vi "panelResize.vi"(4 "error in (no error)":errorcluster, 5 "NewBnds":T1, 7 "control refs":T2) -> (0 "error out":errorcluster)   [LabVIEW 2017]
uses:
  <vilib>/Utility/miscctls.llb/LVRectTypeDef.ctl
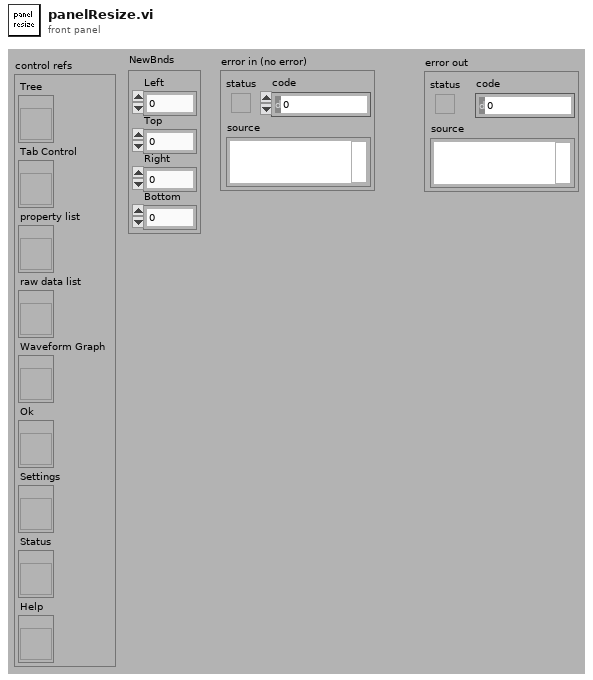
[diagram p1: front panel]
types:
  T1 = typedef "LVRectTypeDef.ctl" = cluster{"Left":i16, "Top":i16, "Right":i16, "Bottom":i16}
  T2 = cluster{"Tree":refnum<vi>, "Tab Control":refnum<vi>, "property list":refnum<vi>, "raw data list":refnum<vi>, "Waveform Graph":refnum<vi>, "Ok":refnum<vi>, "Settings":refnum<vi>, "Status":refnum<vi>, "Help":refnum<vi>}
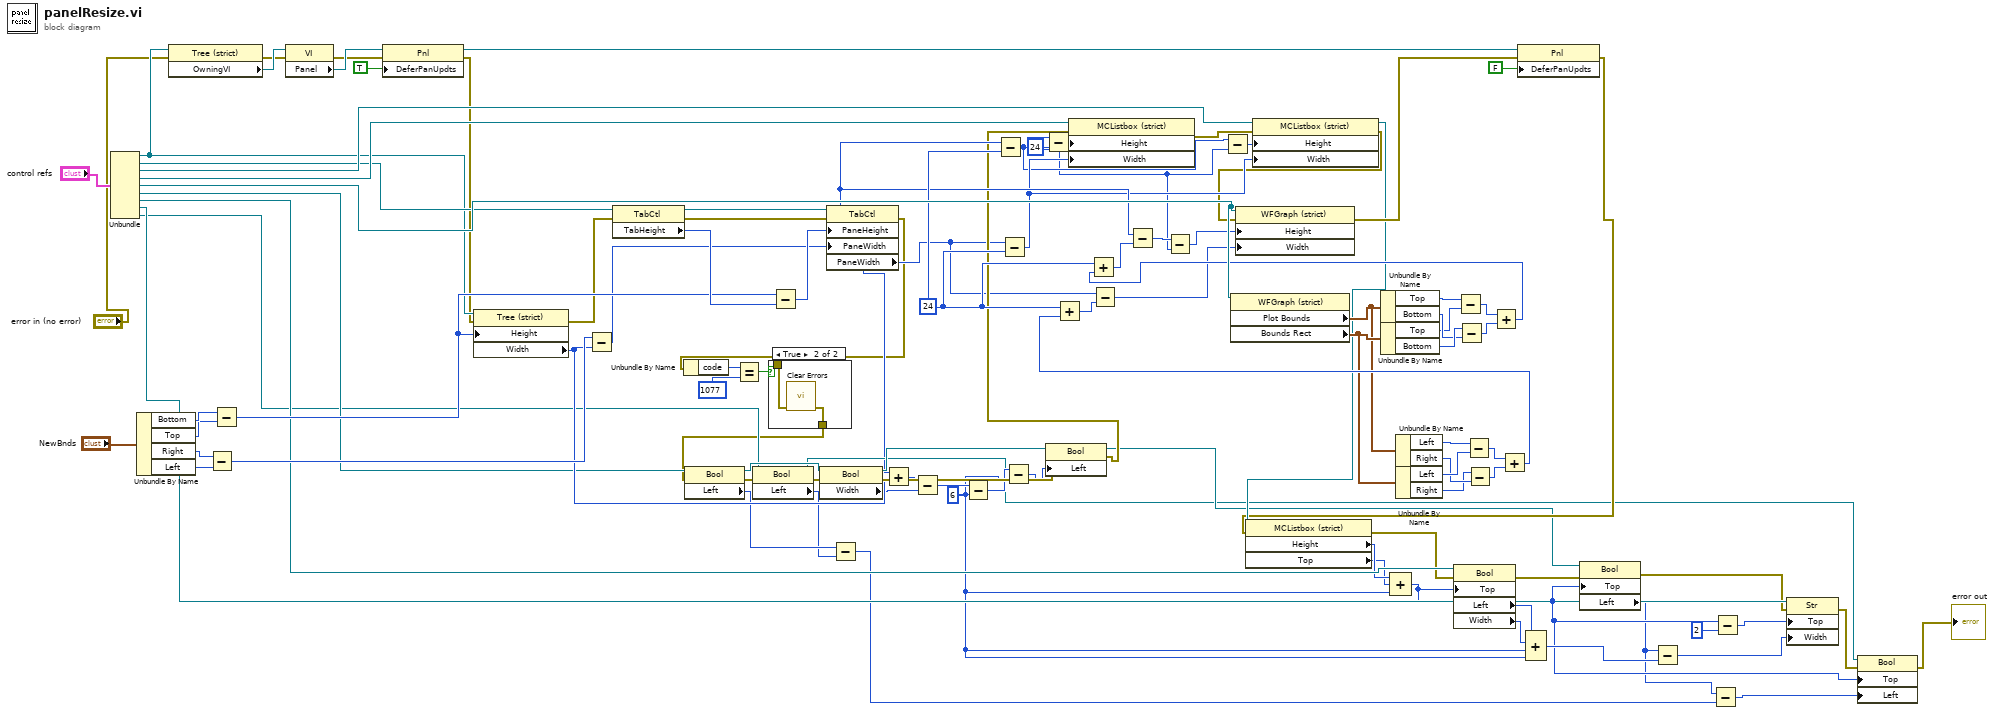
[diagram p0: block diagram]
diagram:
  w42 = u32 24 ("y")
  w23 = u32 6 ("y")
  w92 = u32 24 ("y")
  n1 = Unbundle("control refs") -> ("Tree"=w62:refnum<vi>, "Tab Control"=w101:refnum<vi>, "property list"=w102:refnum<vi>, "raw data list"=w103:refnum<vi>, "Waveform Graph"=w104:refnum<vi>, "Ok"=w22:refnum<vi>, "Settings"=w50:refnum<vi>, "Status"=w33:refnum<vi>, "Help"=w20:refnum<vi>)
  n2 = Unbundle By Name("NewBnds") -> ("Bottom"=w69:i16, "Top"=w68:i16, "Right"=w98:i16, "Left"=w95:i16)
  n3 = property class="Tree (strict)"(reference=w62, error in="error in (no error)") -> (error out=w59:errorcluster, "OwningVI"=w61:refnum<vi>)  [unwired: 1 out]
  n4 = Subtract(x=w98, y=w95) -> (x-y=w96:i16)
  n5 = Subtract(x=w69, y=w68) -> (x-y=w71:i16)
  n6 = property class="VI"(reference=w61, error in=w59) -> (error out=w58:errorcluster, "Panel"=w60:refnum<vi>)  [unwired: 1 out]
  n7 = property class="Pnl"(reference=w60, error in=w58, "DeferPanUpdts"=TRUE ("Defer Panel Updates")) -> (reference out=w54:refnum<vi>, error out=w52:errorcluster)
  n8 = property class="Tree (strict)"(reference=w62, error in=w52, "Height"=w71) -> (error out=w65:errorcluster, "Width"=w51:u32)  [unwired: 1 out]
  n9 = Subtract(x=w96, y=w51) -> (x-y=w7:u32)
  n10 = property class="TabCtl"(reference=w101, error in=w65) -> (reference out=w70:refnum<vi>, error out=w6:errorcluster, "TabHeight"=w72:u32)
  n11 = Subtract(x=w71, y=w72) -> (x-y=w75:u32)
  n12 = property class="TabCtl"(reference=w70, error in=w6, "PaneHeight"=w75, "PaneWidth"=w7) -> (error out=w2:errorcluster, "PaneWidth"=w8:u32)  [unwired: 1 out]
  n13 = Unbundle By Name(w2) -> ("code"=w5:i32)
  n14 = Equal?(x=w5, y=1077) -> (x = y?=w3:bool)
  n15 = case shown="True" w3 {
    tunnel: w2 -> [w105 w107]
    tunnel: [w105 w106] -> w1
    frame False {
    }
    frame True {
      n16 = call <vilib>:"Clear Errors.vi"("error in (no error)"=w107) -> ("error out"=w106:errorcluster)  [unwired: 5 in, 1 out]
    }
  }
  n17 = property class="Bool"(reference=w22, error in=w1) -> (reference out=w21:refnum<vi>, error out=w19:errorcluster, "Left"=w12:i32)
  n18 = property class="Bool"(reference=w20, error in=w19) -> (reference out=w17:refnum<vi>, error out=w18:errorcluster, "Left"=w11:i32)
  n19 = property class="Bool"(reference=w21, error in=w18) -> (reference out=w97:refnum<vi>, error out=w66:errorcluster, "Width"=w48:u32)
  n20 = Subtract(x=w12, y=w11) -> (x-y=w10:i32)
  n21 = Add(x=w8, y=w51) -> (x+y=w49:u32)
  n22 = Subtract(x=w49, y=w48) -> (x-y=w99:u32)
  n23 = Subtract(x=w99, y=w23) -> (x-y=w25:u32)
  n24 = Subtract(x=w75, y=w92) -> (x-y=w43:u32)
  n25 = Subtract(x=w8, y=w92) -> (x-y=w73:u32)
  n26 = Subtract(x=w25, y=w23) -> (x-y=w24:u32)
  n27 = Subtract(x=w43, y=w42) -> (x-y=w45:u32)
  n28 = property class="Bool"(reference=w97, error in=w66, "Left"=w24) -> (reference out=w34:refnum<vi>, error out=w41:errorcluster)
  n29 = property class="MCListbox (strict)"(reference=w103, error in=w41, "Height"=w45, "Width"=w73) -> (error out=w64:errorcluster)  [unwired: 1 out]
  n30 = Subtract(x=w43, y=w42) -> (x-y=w44:u32)
  n31 = property class="WFGraph (strict)"(reference=w104) -> ("Plot Bounds"=w88:T1, "Bounds Rect"=w89:T1)  [unwired: 1 in, 2 out]
  n32 = property class="MCListbox (strict)"(reference=w102, error in=w64, "Height"=w44, "Width"=w73) -> (reference out=w40:refnum<vi>, error out=w63:errorcluster)
  n33 = Unbundle By Name(w88) -> ("Top"=w77:i16, "Bottom"=w78:i16)
  n34 = Unbundle By Name(w89) -> ("Top"=w76:i16, "Bottom"=w79:i16)
  n35 = Unbundle By Name(w88) -> ("Left"=w86:i16, "Right"=w85:i16)
  n36 = Unbundle By Name(w89) -> ("Left"=w87:i16, "Right"=w84:i16)
  n37 = Subtract(x=w77, y=w76) -> (x-y=w80:i16)
  n38 = Subtract(x=w79, y=w78) -> (x-y=w81:i16)
  n39 = Subtract(x=w86, y=w87) -> (x-y=w83:i16)
  n40 = Subtract(x=w84, y=w85) -> (x-y=w82:i16)
  n41 = Add(x=w80, y=w81) -> (x+y=w93:i16)
  n42 = Add(x=w92, y=w93) -> (x+y=w94:u32)
  n43 = Subtract(x=w75, y=w94) -> (x-y=w47:u32)
  n44 = Subtract(x=w47, y=w42) -> (x-y=w46:u32)
  n45 = Add(x=w83, y=w82) -> (x+y=w90:i16)
  n46 = Add(x=w92, y=w90) -> (x+y=w91:u32)
  n47 = Subtract(x=w8, y=w91) -> (x-y=w74:u32)
  n48 = property class="WFGraph (strict)"(reference=w104, error in=w63, "Height"=w46, "Width"=w74) -> (error out=w53:errorcluster)  [unwired: 1 out]
  n49 = property class="Pnl"(reference=w54, error in=w53, "DeferPanUpdts"=FALSE ("Defer Panel Updates")) -> (error out=w38:errorcluster)  [unwired: 1 out]
  n50 = property class="MCListbox (strict)"(reference=w40, error in=w38) -> (error out=w39:errorcluster, "Height"=w37:u32, "Top"=w36:i32)  [unwired: 1 out]
  n51 = Compound Arithmetic op=ADD(w37, w36, w23) -> (w14:u32)
  n52 = property class="Bool"(reference=w50, error in=w39, "Top"=w14) -> (error out=w35:errorcluster, "Left"=w30:i32, "Width"=w31:u32)  [unwired: 1 out]
  n53 = Compound Arithmetic op=ADD(w30, w31, w23, w23) -> (w29:u32)
  n54 = property class="Bool"(reference=w34, error in=w35, "Top"=w14) -> (error out=w32:errorcluster, "Left"=w13:i32)  [unwired: 1 out]
  n55 = Subtract(x=w13, y=w29) -> (x-y=w28:u32)
  n56 = Subtract(x=w13, y=w10) -> (x-y=w9:i32)
  n57 = Subtract(x=w14, y=u32 2) -> (x-y=w27:u32)
  n58 = property class="Str"(reference=w33, error in=w32, "Top"=w27, "Width"=w28) -> (error out=w16:errorcluster)  [unwired: 1 out]
  n59 = property class="Bool"(reference=w17, error in=w16, "Top"=w14, "Left"=w9) -> (error out=→"error out":errorcluster)  [unwired: 1 out]
